vi "DFD Plot Freq Response.vi"   [LabVIEW 2017, in "NI_DigFilterLicensed.lvlib"]
doc: "Plots the frequency responses, including the magnitude and phase responses, of a filter."
uses:
  <vilib>/addons/Digital Filter Design/NI_DigFilterLicensed.lvlib
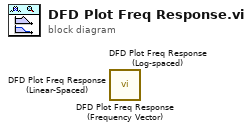
[diagram p0: block diagram]
diagram:
  n1 = call <vilib>:"DFD Plot Freq Response (Frequency Vector).vi"() -> ()  [unwired: 8 in, 4 out]
  n2 = call <vilib>:"DFD Plot Freq Response (Log-spaced).vi"() -> ()  [unwired: 8 in, 4 out]
  n3 = call <vilib>:"DFD Plot Freq Response (Linear-Spaced).vi"() -> ()  [unwired: 8 in, 4 out]
